vi "CO Air Free Percentage Limit Check.vi"(10 "54-55 Minutes CO Air Free":dbl[](array[numeric]), 11 "24-25 Minutes CO Air Free":dbl[](array[numeric])) -> (3 "CO Air Free In Spec":bool)   [LabVIEW 2023]
uses:
  <vilib>/Analysis/baseanly.llb/Mean (DBL).vi
  <vilib>/Analysis/NI_AALBase.lvlib
panel:
  out "24-25 Minutes CO Air Free - Upper Limit":dbl
  out "54-55 Minutes CO Air Free":dbl format="%.8f"
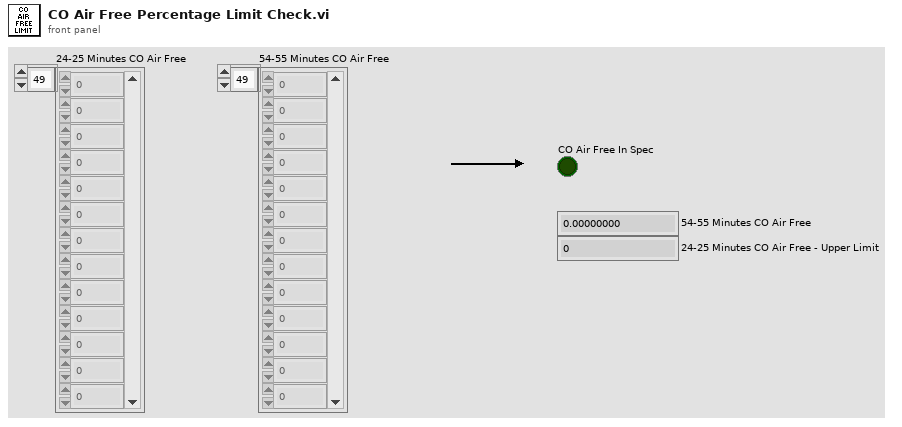
[diagram p1: front panel]
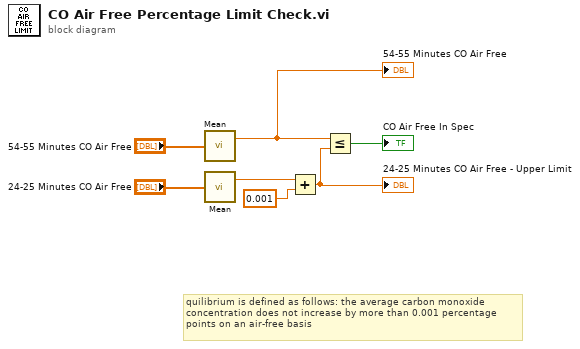
[diagram p0: block diagram]
diagram:
  # "quilibrium is defined as follows: the average carbon monoxide\nconcentration does not increase by more than 0.001 percentage\npoints on an air-free basis"
  n1 = call-poly <vilib>:"Mean.vi"("X"="54-55 Minutes CO Air Free") -> ("mean"=w7:dbl)  [unwired: 1 out]
  "54-55 Minutes CO Air Free" <- w7
  n2 = call-poly <vilib>:"Mean.vi"("X"="24-25 Minutes CO Air Free") -> ("mean"=w3:dbl)  [unwired: 1 out]
  n3 = Add(x=w3, y=0.001) -> (x+y=w5:dbl)
  "24-25 Minutes CO Air Free - Upper Limit" <- w5
  n4 = Less Or Equal?(x=w7, y=w5) -> (x <= y?=→"CO Air Free In Spec":bool)
